vi "Photo Get Luminous Intensity.vi"(8 "error in (no error)":errorcluster, 9 "a_distancecm":dbl, 10 "a_CIEResolution":u8, 11 "a_data":dbl[](array[numeric])) -> (0 "error out":errorcluster, 2 "function return":i16, 3 "a_data out":dbl[](array[numeric]), 5 "a_Candela out":dbl)   [LabVIEW 2013, in "AVSirrad.lvlib"]
doc: "DLL_API short int __stdcall Photo_GetLuminousIntensity\n( \n DataType *a_data,\n unsigned char a_CIEResolution,\n double a_distancecm,\n double *a_Candela\n);"
uses:
  AVSirrad.lvlib
  AVSIRRAD/Examples/Labview/build/AVSirrad.dll
panel:
  in  "a_Candela":dbl
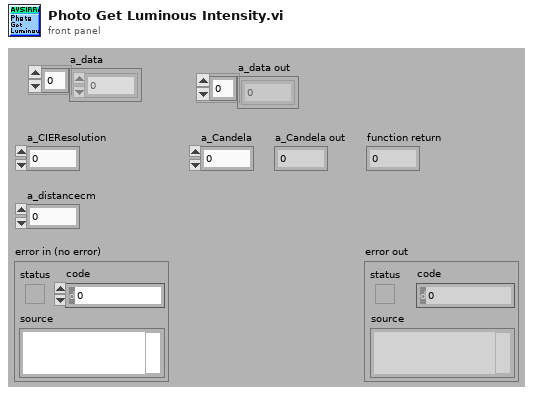
[diagram p1: front panel]
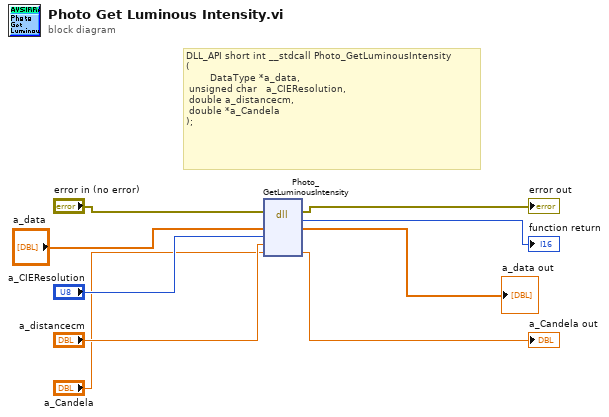
[diagram p0: block diagram]
diagram:
  # "DLL_API short int __stdcall Photo_GetLuminousIntensity\n( \n        DataType *a_data,\n\tunsigned char   a_CIEResolution,\n\tdouble a_distancecm,\n\tdouble *a_Candela\n);"
  n1 = dll-call lib="C:/AVSIRRAD/Examples/Labview/build/AVSirrad.*" fn="Photo_GetLuminousIntensity"(error in="error in (no error)", "a_data"="a_data", "a_CIEResolution"="a_CIEResolution", "a_distancecm"="a_distancecm", "a_Candela"="a_Candela") -> (error out=→"error out":errorcluster, "return type"=→"function return":i16, "a_data"=→"a_data out":dbl[], "a_Candela"=→"a_Candela out":dbl)  [unwired: 4 in, 1 out]
